vi "Initialize.vi"(0 "ACM4509 in":refnum<class "Cal Standard.lvclass">, 11 "error in (no error)":errorcluster) -> (4 "ACM4509 out":refnum<class "Cal Standard.lvclass">, 6 "Found":bool, 15 "error out":errorcluster)   [LabVIEW 2023, in "ACM 4509 Cal Standard.lvlib" / "Cal Standard.lvclass"]
uses:
  Cal Standard.lvclass
  C:/srd-semi-rfcal-software/AuxTools/STSRFFixtureCharactUtility/Source/Code Modules/Fixture/Instruments/Cal Standard/Cal Standard Base/Cal Standard Base.lvclass
  Cal Standard.lvclass/Cal Standard.ctl
  Instruments/Cal Standard/Cal Standard Base/Cal Standard Base.lvclass/Cal Standard Base.ctl
  Properties/Write Resource Name.vi
  Instruments/Cal Standard/Cal Standard Base/Properties/Write Instrument Info.vi
  Instruments/Cal Standard/Cal Standard Base/Properties/Write Path Connection Map.vi
  <vilib>/nisyscfg/Find Hardware.vi
  <vilib>/nisyscfg/Close (System).vi
  <vilib>/nisyscfg/nisyscfg.lvlib
  <resource>/objmgr/rfSysapiTags.rc
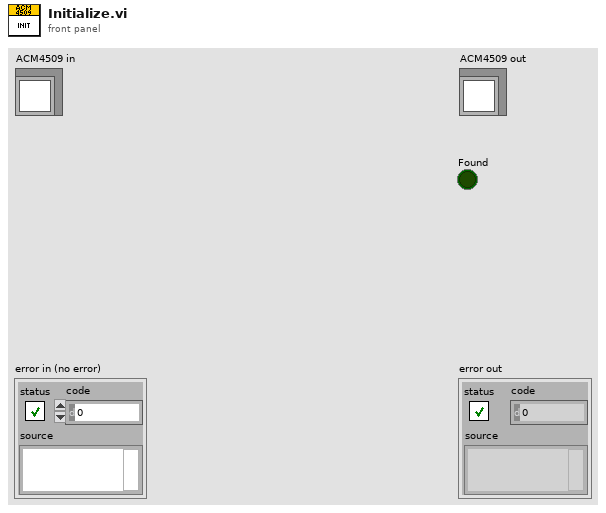
[diagram p1: front panel]
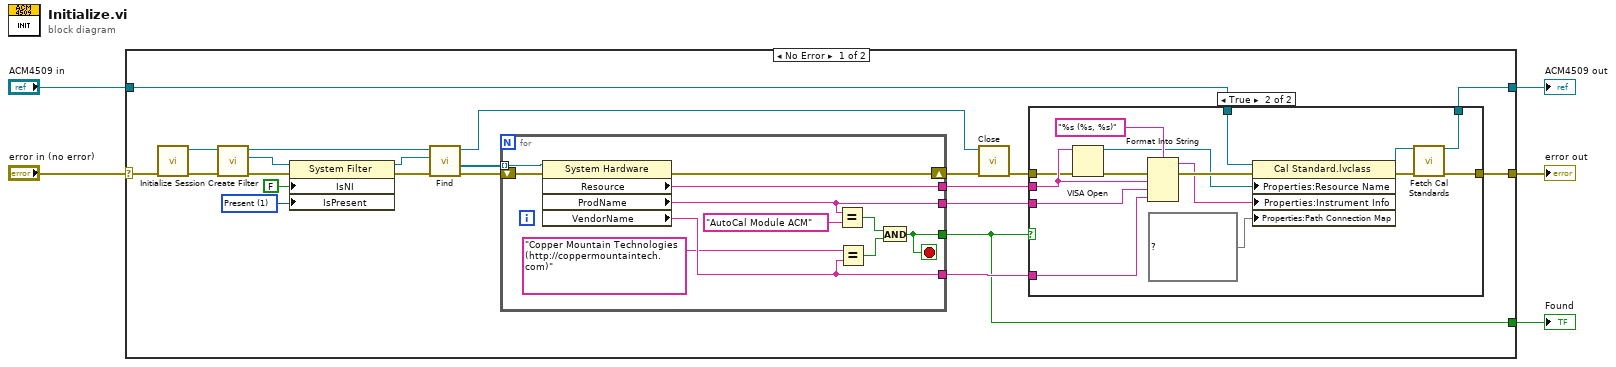
[diagram p0: block diagram]
diagram:
  n1 = case shown="No Error" "error in (no error)" {
    selector: "error in (no error)" -> [w17 w57]
    tunnel: [w7 w57] -> w4
    tunnel: "ACM4509 in" -> [w16 w56]
    tunnel: [w15 w56] -> w3
    tunnel: [w6 _] -> w1
    frame No Error {
      w19 = 1 items=["Unknown"=-1, "Not Present"=0, "Present"=1] ("Devices & Chassis:Is Present")
      n2 = call <vilib>:"Initialize Session.vi"("error in (no error)"=w17) -> ("error out"=w18:errorcluster, "Session out"=w20:refnum<k21>)  [unwired: 9 in]
      n3 = call <vilib>:"Create Filter.vi"("error in (no error)"=w18, "Session in"=w20) -> ("error out"=w26:errorcluster, "Filter out"=w25:refnum<k20>, "Session out"=w23:refnum<k21>)  [unwired: 7 in]
      n4 = property class="System Filter"(reference=w25, error in=w26, "IsNI"=FALSE ("Devices & Chassis:Is NI Product"), "IsPresent"=w19) -> (reference out=w24:refnum<k20>, error out=w22:errorcluster)
      n5 = call-poly <vilib>:"Find.vi"("error in (no error)"=w22, "Filter in"=w24, "Session in"=w23) -> ("error out"=w27:errorcluster, "Resources out"=w14:refnum<k20>[], "Session out"=w8:refnum<k21>)  [unwired: 5 in, 1 out]
      n6 = for {
        tunnel: [w52] -> w13
        tunnel: [w53] -> w12
        shift-right: [w54] -> w10
        shift-left: w27 -> [w55]
        tunnel: [w49] -> w11
        tunnel: w14 -> [w46] mode=indexing
        tunnel: [w45] -> w6
        stop <- w45 stop-if-true
        n7 = property class="System Hardware"(reference=w46, error in=w55) -> (error out=w54:errorcluster, "Resource"=w53:string, "ProdName"=w52:string, "VendorName"=w49:string)  [unwired: 1 out]
        n8 = Equal?(x=w52, y="AutoCal Module ACM") -> (x = y?=w50:bool)
        n9 = Equal?(x="Copper Mountain Technologies (http://coppermountaintech.com)", y=w49) -> (x = y?=w47:bool)
        n10 = And(x=w50, y=w47) -> (x .and. y?=w45:bool)
      }
      n11 = call-poly <vilib>:"Close.vi"("error in (no error)"=w10, "Session in"=w8) -> ("error out"=w9:errorcluster)  [unwired: 9 in]
      n12 = case shown="True" w6 {
        tunnel: w16 -> [w28 w44]
        tunnel: [w28 w32] -> w15
        tunnel: [w29 w34] -> w7
        tunnel: w13 -> [_ w41]
        tunnel: w12 -> [_ w39]
        tunnel: w11 -> [_ w37]
        tunnel: w9 -> [w29 w36]
        frame False {
        }
        frame True {
          n13 = VISA Open(error in (no error)=w36, VISA resource name=w39) -> (VISA resource name=w38:refnum<visa-resource-name>, error out=w40:errorcluster)  [unwired: 3 in]
          n14 = Format Into String(format string="%s (%s, %s)", error in=w40, w39, w41, w37) -> (resulting string=w31:string, error out=w42:errorcluster)  [unwired: 1 in]
          n15 = property class="Cal Standard.lvclass"(reference=w44, error in=w42, "Properties:Resource Name"=w38, "Properties:Instrument Info"=w31, "Properties:Path Connection Map"=map{string, string[]} {} ("Path Connection Map")) -> (reference out=w33:refnum<class "Cal Standard.lvclass">, error out=w35:errorcluster)
          n16 = call "Fetch Cal Standards.vi"("ACM4509 in"=w33, "error in (no error)"=w35) -> ("ACM4509 out"=w32:refnum<class "Cal Standard.lvclass">, "error out"=w34:errorcluster)  [unwired: 12 in]
        }
      }
    }
    frame Error {
    }
  }
  "error out" <- w4
  "ACM4509 out" <- w3
  "Found" <- w1
